vi "Error_Classifier.vi"(0 "PSRR":i32, 11 "Error in":errorcluster) -> (2 "Error?":bool, 3 "PSRR":i32(graph), 4 "Error Code":i32, 6 "Description":string, 8 "Type":string, 10 "Stop":bool, 15 "Error out":errorcluster)   [LabVIEW 2020]
doc: "This VI is used to classify different errors and give the results to the PSRR monitor"
uses:
  Typedefs/Stop cases.ctl
  Typedefs/LV2 numeric.ctl
panel:
  out "Error des":string
  in  "Warning":dbl
  in  "Passive error":dbl
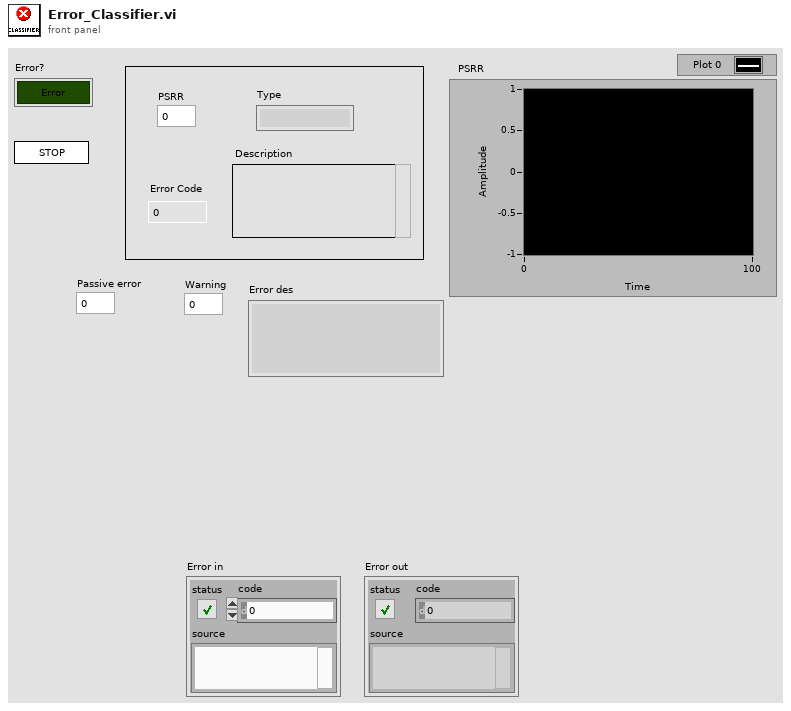
[diagram p1: front panel]
types:
  T1 = typedef "LV2 numeric.ctl" = enum16{"Initialize", "Read", "Write"}
  T2 = typedef "Stop cases.ctl" = enum16{"Initialize", "Write", "Stop"}
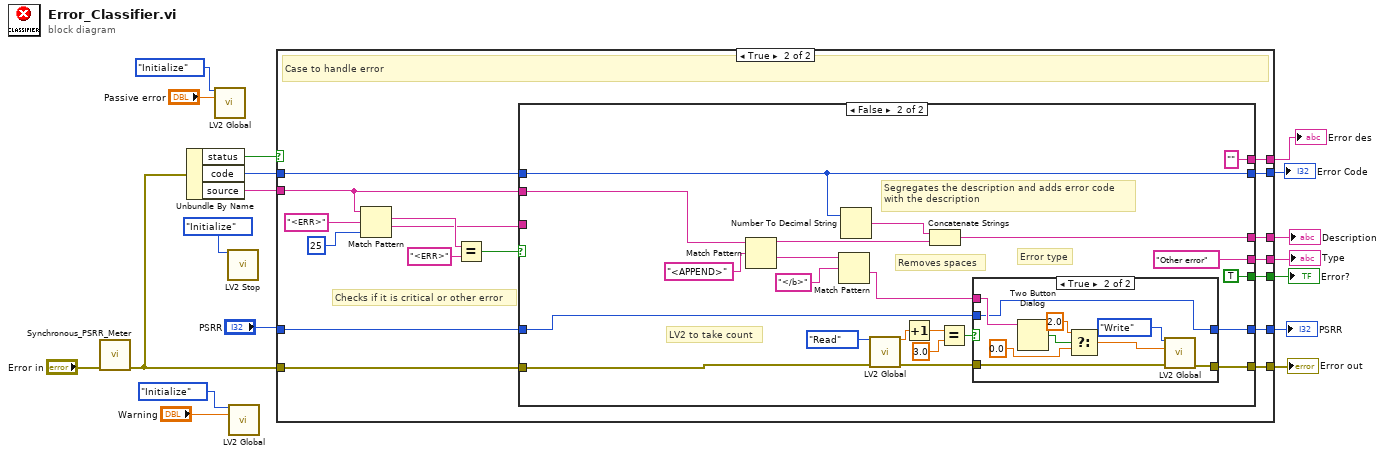
[diagram p0: block diagram]
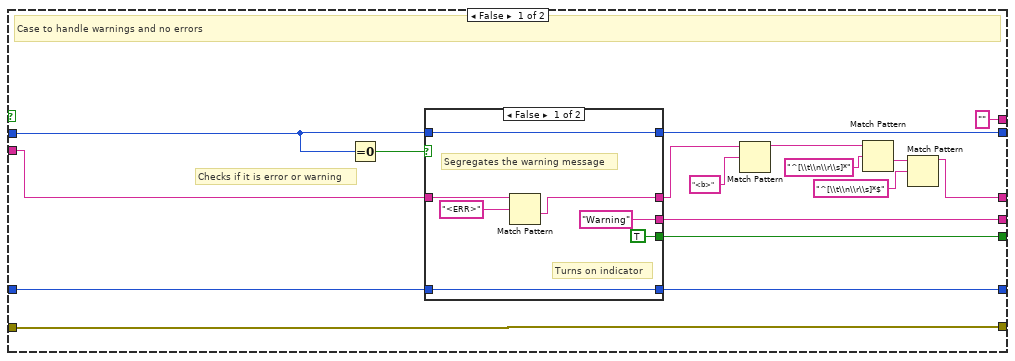
[diagram p2: hidden frame]
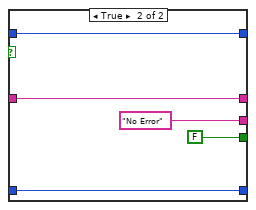
[diagram p3: hidden frame]
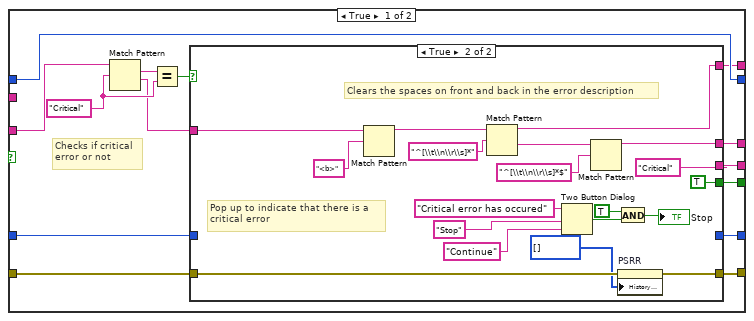
[diagram p4: hidden frame]
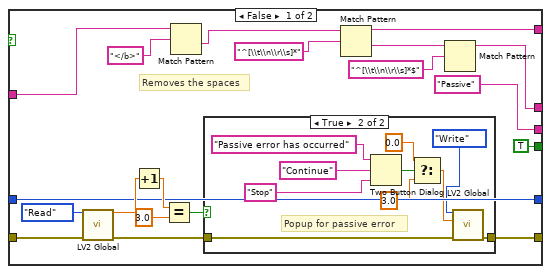
[diagram p5: hidden frame]
diagram:
  n1 = call "Synchronous_PSRR_Meter.vi"("error in"="Error in") -> ("error out"=w2:errorcluster)  [unwired: 9 in, 1 out]
  n2 = Unbundle By Name(w2) -> ("status"=w16:bool, "code"=w14:i32, "source"=w15:string)
  n3 = call "LV2 Global.vi"("Operation"=LV2_numeric."Initialize", "Numeric Input"="Passive error") -> ()  [unwired: 12 in, 2 out]
  n4 = call "LV2 Stop.vi"("Operation"=Stop_cases."Initialize") -> ()  [unwired: 13 in, 2 out]
  n5 = call "LV2 Global.vi"("Operation"=LV2_numeric."Initialize", "Numeric Input"="Warning") -> ()  [unwired: 12 in, 2 out]
  n6 = case shown="True" w16 {
    tunnel: w15 -> [w35 w57]
    tunnel: [w19 w58] -> w18
    tunnel: w14 -> [w27 w56]
    tunnel: "PSRR" -> [w34 w50]
    tunnel: [w33 w49] -> w12
    tunnel: [w31 w55] -> w11
    tunnel: [w30 w54] -> w10
    tunnel: [w28 w53] -> w9
    tunnel: [w29 w52] -> w8
    tunnel: w2 -> [w29 w51]
    tunnel: ["" ("source") w48] -> w1
    frame False {
      # "Checks if it is error or warning"
      # "Case to handle warnings and no errors"
      n7 = Equal To 0?(x=w27) -> (x = 0?=w32:bool)
      n8 = case shown="False" w32 {
        tunnel: w35 -> [w40 w47]
        tunnel: [w36 w47] -> w20
        tunnel: w34 -> [w42 w46]
        tunnel: [w42 w46] -> w33
        tunnel: ["Warning" "No Error"] -> w31
        tunnel: [TRUE ("Error?") FALSE ("Error?")] -> w30
        tunnel: [w37 w43] -> w28
        tunnel: w27 -> [w37 w43]
        frame False {
          # "Turns on indicator"
          # "Segregates the warning message"
          n9 = Match Pattern(string=w40, regular expression="<ERR>") -> (after substring=w36:string)  [unwired: 1 in, 3 out]
        }
        frame True {
        }
      }
      n10 = Match Pattern(string=w20, regular expression="<b>") -> (before substring=w21:string)  [unwired: 1 in, 3 out]
      n11 = Match Pattern(string=w21, regular expression="^[\\t\\n\\r\\s]*") -> (after substring=w25:string)  [unwired: 1 in, 3 out]
      n12 = Match Pattern(string=w25, regular expression="^[\\t\\n\\r\\s]*$") -> (before substring=w19:string)  [unwired: 1 in, 3 out]
    }
    frame True {
      # "Checks if it is critical or other error"
      # "Case to handle error"
      n13 = Match Pattern(string=w57, regular expression="<ERR>", offset (0)=25) -> (match substring=w62:string, after substring=w59:string)  [unwired: 2 out]
      n14 = Equal?(x=w62, y="<ERR>" ("regular expression")) -> (x = y?=w60:bool)
      n15 = case shown="False" w60 {
        tunnel: w59 -> [w73 _]
        tunnel: [w76 w134] -> w58
        tunnel: w57 -> [_ w149]
        tunnel: w56 -> [w69 w136]
        tunnel: [w75 "Other error"] -> w55
        tunnel: [w74 TRUE ("Error?")] -> w54
        tunnel: [w69 w136] -> w53
        tunnel: [w71 w133] -> w52
        tunnel: w51 -> [w72 w131]
        tunnel: w50 -> [w68 w130]
        tunnel: [w67 w129] -> w49
        tunnel: [w66 "" ("source")] -> w48
        frame True {
          w70 = "Critical" ("regular expression")
          # "Checks if critical\nerror or not"
          n16 = Match Pattern(string=w73, regular expression=w70) -> (match substring=w78:string, after substring=w65:string)  [unwired: 1 in, 2 out]
          n17 = Equal?(x=w78, y=w70) -> (x = y?=w77:bool)
          n18 = case shown="True" w77 {
            tunnel: w65 -> [w94 w118]
            tunnel: [w93 w116] -> w76
            tunnel: ["Passive" "Critical"] -> w75
            tunnel: [TRUE ("Error?") TRUE ("Error?")] -> w74
            tunnel: w72 -> [w83 w112]
            tunnel: [w81 w111] -> w71
            tunnel: w68 -> [w80 _]
            tunnel: [w80 _] -> w67
            tunnel: [w79 w109] -> w66
            frame False {
              # "Removes the spaces"
              n19 = call "LV2 Global.vi"("Operation"=LV2_numeric."Read", "Error in"=w83) -> ("Numeric Output"=w85:dbl, "Error out"=w82:errorcluster)  [unwired: 12 in]
              n20 = Increment(x=w85) -> (x+1=w84:dbl)
              n21 = Equal?(x=w84, y=3.0) -> (x = y?=w91:bool)
              n22 = Match Pattern(string=w94, regular expression="</b>") -> (after substring=w86:string)  [unwired: 1 in, 3 out]
              n23 = case shown="True" w91 {
                tunnel: w82 -> [w98 w100]
                tunnel: [w98 w99] -> w81
                frame False {
                }
                frame True {
                  # "Popup for passive error"
                  n24 = Two Button Dialog(message="Passive error has occurred", 1:"Stop" ("F button name (\"Cancel\")"), 2:"Continue" ("T button name (\"OK\")")) -> (T button?=w105:bool)
                  n25 = Select(t=0.0, s=w105, f=3.0) -> (s? t:f=w102:dbl)
                  n26 = call "LV2 Global.vi"("Operation"=LV2_numeric."Write", "Numeric Input"=w102, "Error in"=w100) -> ("Error out"=w99:errorcluster)  [unwired: 11 in, 1 out]
                }
              }
              n27 = Match Pattern(string=w86, regular expression="^[\\t\\n\\r\\s]*") -> (before substring=w79:string, after substring=w96:string)  [unwired: 1 in, 2 out]
              n28 = Match Pattern(string=w96, regular expression="^[\\t\\n\\r\\s]*$") -> (before substring=w93:string)  [unwired: 1 in, 3 out]
            }
            frame True {
              # "Pop up to indicate that there is a \ncritical error"
              # "Clears the spaces on front and back in the error description"
              n29 = Match Pattern(string=w118, regular expression="<b>") -> (before substring=w117:string)  [unwired: 1 in, 3 out]
              n30 = Match Pattern(string=w117, regular expression="^[\\t\\n\\r\\s]*") -> (before substring=w109:string, after substring=w122:string)  [unwired: 1 in, 2 out]
              n31 = Two Button Dialog(message="Critical error has occured", 1:"Continue" ("F button name (\"Cancel\")"), 2:"Stop" ("T button name (\"OK\")")) -> (T button?=w124:bool)
              n32 = Match Pattern(string=w122, regular expression="^[\\t\\n\\r\\s]*$") -> (before substring=w116:string)  [unwired: 1 in, 3 out]
              n33 = And(x=TRUE, y=w124) -> (x .and. y?=→"Stop":bool)
              n34 = property on="PSRR" class="WFChart (strict)"(error in=w112, "History Data"=i32[] []) -> (error out=w111:errorcluster)  [unwired: 1 in, 1 out]
            }
          }
        }
        frame False, Default {
          # "Error type"
          # "LV2 to take count"
          # "Removes spaces"
          # "Segregates the description and adds error code \nwith the description"
          n35 = Match Pattern(string=w149, regular expression="<APPEND>") -> (before substring=w146:string, after substring=w145:string)  [unwired: 1 in, 2 out]
          n36 = Match Pattern(string=w145, regular expression="</b>") -> (after substring=w139:string)  [unwired: 1 in, 3 out]
          n37 = Number To Decimal String(number=w136) -> (decimal integer string=w147:string)  [unwired: 1 in]
          n38 = call "LV2 Global.vi"("Operation"=LV2_numeric."Read", "Error in"=w131) -> ("Numeric Output"=w142:dbl, "Error out"=w132:errorcluster)  [unwired: 12 in]
          n39 = Increment(x=w142) -> (x+1=w135:dbl)
          n40 = Concatenate Strings(w147, w146) -> (w134:string)
          n41 = Equal?(x=w135, y=3.0) -> (x = y?=w140:bool)
          n42 = case shown="True" w140 {
            tunnel: w139 -> [_ w160]
            tunnel: [w151 w154] -> w133
            tunnel: w132 -> [w151 w153]
            tunnel: w130 -> [w150 w152]
            tunnel: [w150 w152] -> w129
            frame False {
            }
            frame True {
              n43 = Two Button Dialog(message=w160) -> (T button?=w157:bool)  [unwired: 2 in]
              n44 = Select(t=2.0, s=w157, f=0.0) -> (s? t:f=w158:dbl)
              n45 = call "LV2 Global.vi"("Operation"=LV2_numeric."Write", "Numeric Input"=w158, "Error in"=w153) -> ("Error out"=w154:errorcluster)  [unwired: 11 in, 1 out]
            }
          }
        }
      }
    }
  }
  "Description" <- w18
  "Error out" <- w8
  "PSRR" <- w12
  "Type" <- w11
  "Error?" <- w10
  "Error Code" <- w9
  "Error des" <- w1
